vi "Test To and From Binary for Functions.vi"() -> ()   [LabVIEW 2021]
uses:
  Source/Abs_Types/Double Float/Support/Type.ctl
  Source/Functions/Support/Function/Two Terminal/DBL/AbsFunc_Two Term_DBL.lvclass
  Source/Constants/Support/DBL/Const_DBL.lvclass
  C:/TSA/LV_Abstract/Source/Abs_Types/Double Float/Abs_Double Float.lvclass
  C:/Program Files (x86)/National Instruments/LabVIEW 2021/vi.lib/TSA/Abstract Data Classes/Abs_Types/Numeric/Abs_Numeric.lvclass
  Source/Functions/Math/Support/Subtract/DBL/Method.vi
  Source/Abs_Types/Double Float/Abs_Double Float.lvclass
  Source/Functions/Math/Support/Subtract/DBL/Subtract_DBL.lvclass
  C:/TSA/LV_Abstract/Source/Abs_Types/Floating Point/Abs_Floating Point.lvclass
  C:/Program Files (x86)/National Instruments/LabVIEW 2021/vi.lib/TSA/Abstract Data Classes/Abs_Types/Value/Abs_Value.lvclass
  C:/Program Files (x86)/National Instruments/LabVIEW 2021/vi.lib/TSA/Abstract Data Classes/Abs_Types/Type/Abs_Type.lvclass
  C:/TSA/LV_Abstract/Source/Constants/Support/DBL/Const_DBL.lvclass
panel:
  out "Remaning Binary":string
  out "Numeric":dbl
  out "Binary":string
  out "Value":T1
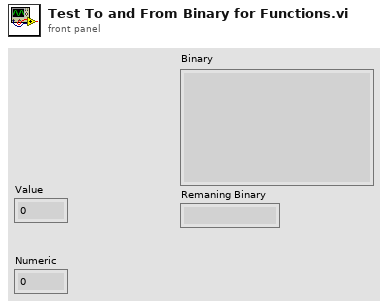
[diagram p1: front panel]
types:
  T1 = typedef "Abs_Double Float.lvclass/Type.ctl" = dbl
  T2 = typedef "Subtract_DBL.lvclass/Abs Type.ctl" = refnum<class "Abs_Double Float.lvclass">
  T3 = typedef "AbsFunc_Two Term_DBL.lvclass/Data Type.ctl" = dbl
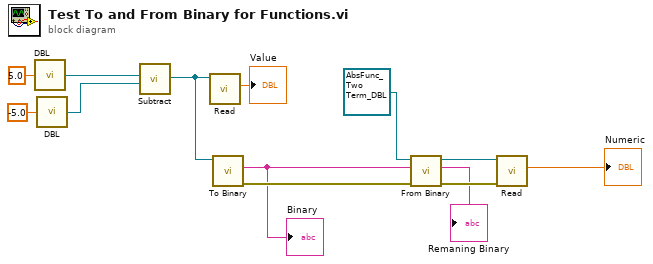
[diagram p0: block diagram]
diagram:
  n1 = call "DBL.vi"("Value"=5.0 ("Numeric")) -> ("Constant"=w13:refnum<class "Const_DBL.lvclass">)  [unwired: 4 in]
  n2 = call "DBL.vi"("Value"=-5.0 ("Numeric")) -> ("Constant"=w12:refnum<class "Const_DBL.lvclass">)  [unwired: 4 in]
  n3 = call-poly "Subtract.vi"("Input B"=w12, "Input A"=w13) -> ("Result"=w8:T2)  [unwired: 4 in]
  n4 = call-dynamic "Read.vi"("Double Float.lvclass_340760 in"=w8) -> ("Value"=→"Value":T1)  [unwired: 8 in, 2 out]
  n5 = call-dynamic "To Binary.vi"("Double Float in"=w8) -> ("error out"=w7:errorcluster, "Binary"=w1:string)  [unwired: 8 in, 1 out]
  "Binary" <- w1
  n6 = call-dynamic "From Binary.vi"("error in (no error)"=w7, "Binary"=w1, "Double Float in"=refnum<class "AbsFunc_Two Term_DBL.lvclass"> refnum ("AbsFunc_Two Term_DBL.lvclass")) -> ("error out"=w6:errorcluster, "Remaining"=→"Remaning Binary":string, "Double Float out"=w5:refnum<class "AbsFunc_Two Term_DBL.lvclass">)  [unwired: 6 in]
  n7 = call-dynamic "Read.vi"("error in (no error)"=w6, "Add in"=w5) -> ("Numeric"=→"Numeric":T3)  [unwired: 7 in, 2 out]
